vi "Lian_Conditional_Statistics.vi"() -> ()   [LabVIEW 2020]
uses:
  <vilib>/numeric/Random Number (Range) U64.vi
  <vilib>/numeric/sub_Random U32.vi
  <vilib>/Analysis/NI_AALBase.lvlib
panel:
  out "Final Array":u64[](array[numeric])
  out "Histogram":T1(graph)
  out "Mean":dbl
  out "Std Dev":dbl
  out "Final Array Size":i32
  out "Iteration Count":i32
  in  "Array Length":i32=100
  out "Final Array Size":i32
  out "Std Dev":dbl
  out "Mean":dbl
  out "FInal Array":dbl[](array[numeric])
  out "Histogram":T1(graph)
  in  "Array Length":i32=100
  in  "?":bool
  out "Iteration Count":i32
  out "Final Array Size":i32
  out "Iteration Count":i32
  out "Std Dev":dbl
  out "Mean":dbl
  out "FInal Array":dbl[](array[numeric])
  in  "?":bool
  out "Histogram":T1(graph)
  in  "Array Length":i32=100
  # "Conditional Statistics"
  # "Description: Filters data using logic and builds array"
  # "Conditional Statistics 3"
  # "Description:  Builds array with select data"
  # "Conditional Statistics 2"
  # "Description: Filters data using selector label and builds array"
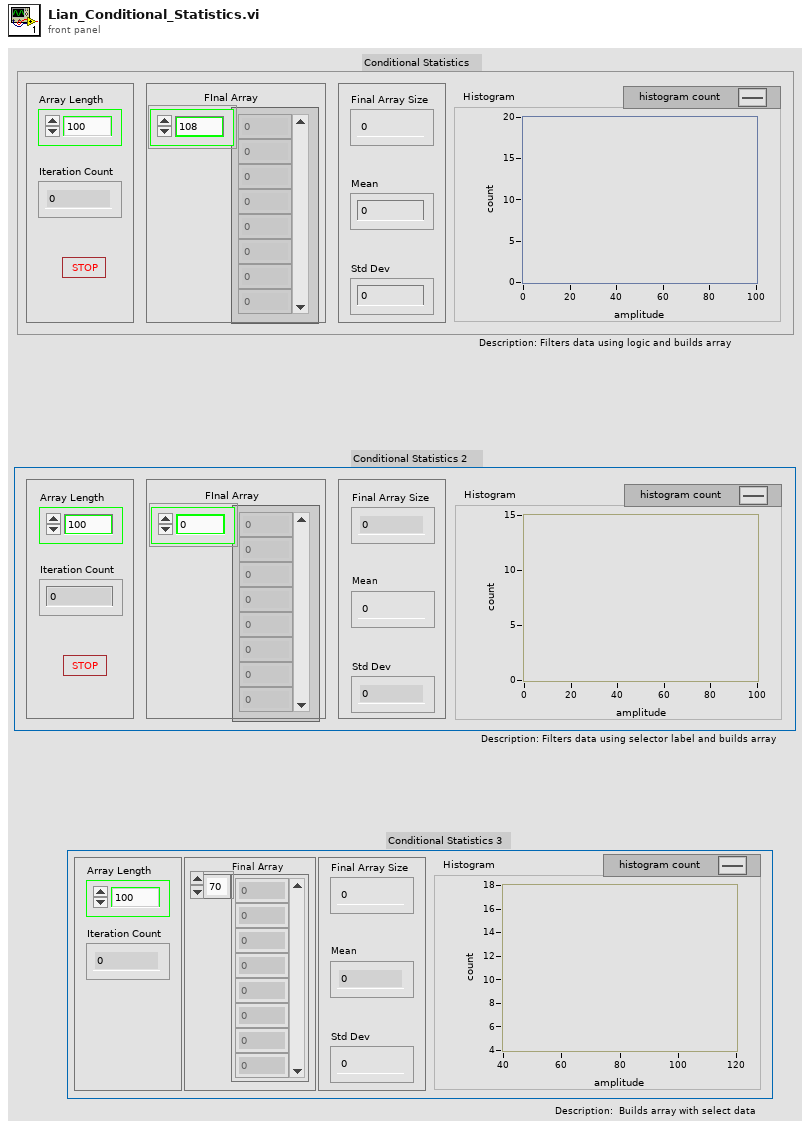
[diagram p1: front panel]
types:
  T1 = cluster{"X Values":dbl[], "Histogram: h(x)":i32[]}
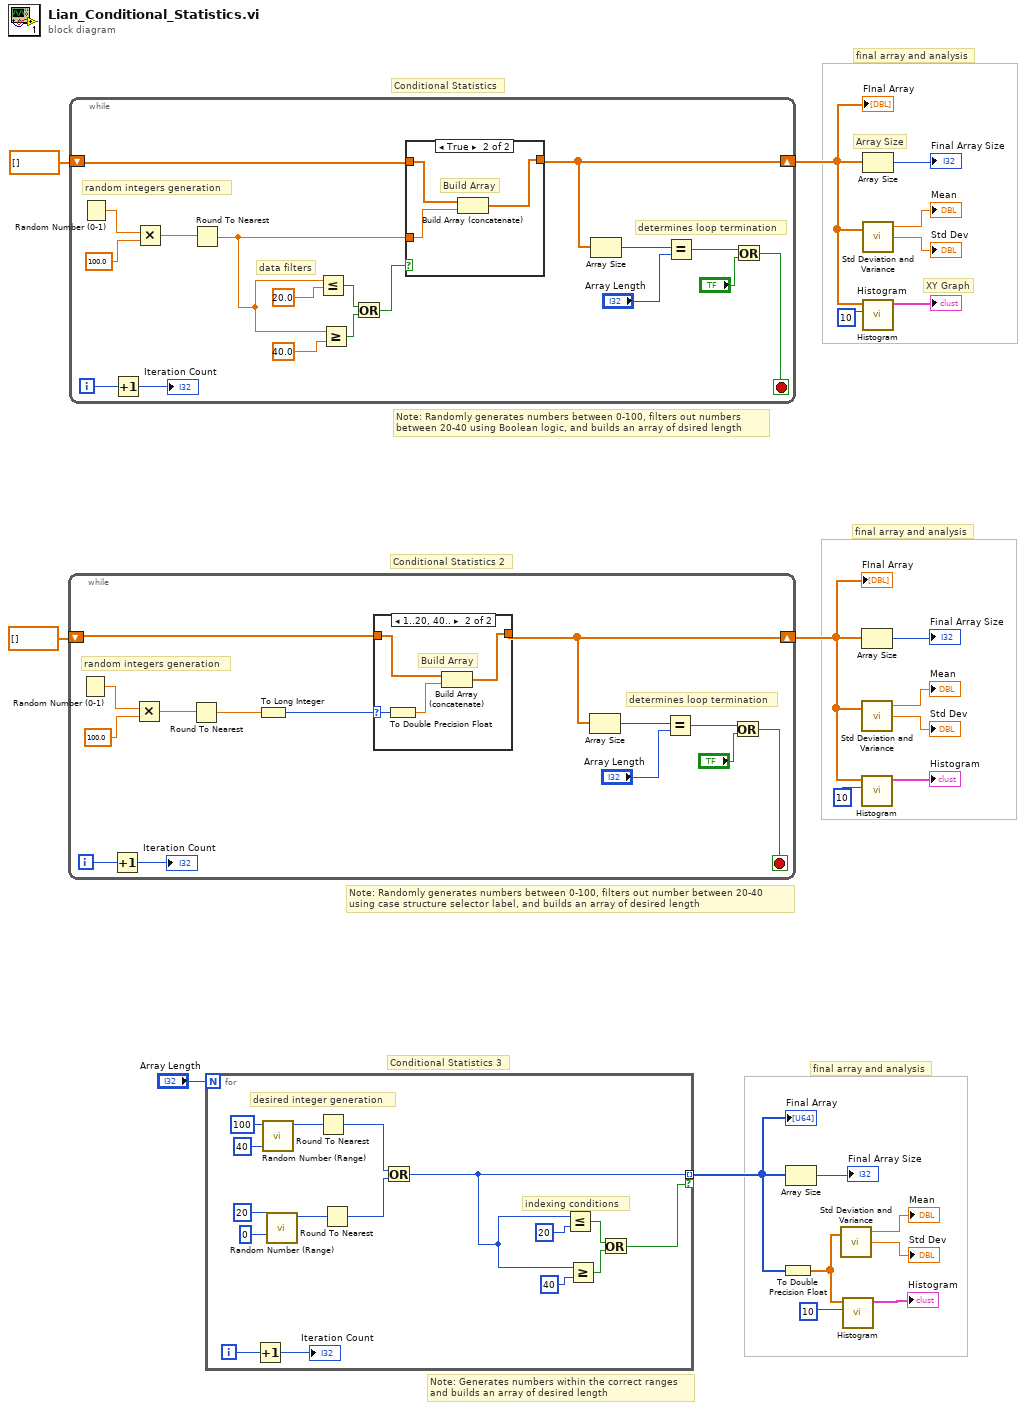
[diagram p0: block diagram]
diagram:
  # "Note: Generates numbers within the correct ranges\nand builds an array of desired length"
  # "Conditional Statistics 3"
  # "final array and analysis"
  # "Array Size"
  # "XY Graph"
  # "Note: Randomly generates numbers between 0-100, filters out number between 20-40 \nusing case structure selector label, and builds an array of desired length"
  # "Conditional Statistics 2"
  # "final array and analysis"
  # "Note: Randomly generates numbers between 0-100, filters out numbers \nbetween 20-40 using Boolean logic, and builds an array of dsired length"
  # "Conditional Statistics"
  # "final array and analysis"
  n1 = while {
    shift-right: [w28] -> w13
    shift-left: dbl[] [] -> [w29]
    i -> [w27]
    stop <- w33 stop-if-true
    # "determines loop termination"
    # "random integers generation"
    n2 = Random Number (0-1)() -> (number: 0 to 1=w36:dbl)
    n3 = Increment(x=w27) -> (x+1=→"Iteration Count":i32)
    n4 = Multiply(x=w36, y=100.0) -> (x*y=w34:dbl)
    n5 = Round To Nearest(number=w34) -> (nearest integer value=w24:dbl)
    n6 = To Long Integer(number=w24) -> (32bit integer=w23:i32)
    n7 = case shown="1..20, 40.." w23 {
      selector: w23 -> [_ w39]
      tunnel: w29 -> [w37 w41]
      tunnel: [w37 w40] -> w28
      frame 21..39, Default {
      }
      frame 1..20, 40.. {
        # "Build Array"
        n8 = To Double Precision Float(number=w39) -> (double precision float=w38:dbl)
        n9 = Build Array (concatenate)(w41, w38) -> (w40:dbl[])
      }
    }
    n10 = Array Size(array=w28) -> (size(s)=w32:i32)
    n11 = Equal?(x=w32, y="Array Length") -> (x = y?=w31:bool)
    n12 = Or(x=w31, y="?") -> (x .or. y?=w33:bool)
  }
  "FInal Array" <- w13
  n13 = while {
    shift-right: [w51] -> w20
    shift-left: dbl[] [] -> [w52]
    i -> [w44]
    stop <- w56 stop-if-true
    # "determines loop termination"
    # "random integers generation"
    # "data filters"
    n14 = Random Number (0-1)() -> (number: 0 to 1=w59:dbl)
    n15 = Increment(x=w44) -> (x+1=→"Iteration Count":i32)
    n16 = Multiply(x=w59, y=100.0) -> (x*y=w57:dbl)
    n17 = Round To Nearest(number=w57) -> (nearest integer value=w47:dbl)
    n18 = Less Or Equal?(x=w47, y=20.0) -> (x <= y?=w50:bool)
    n19 = Greater Or Equal?(x=w47, y=40.0) -> (x >= y?=w49:bool)
    n20 = Or(x=w50, y=w49) -> (x .or. y?=w48:bool)
    n21 = case shown="True" w48 {
      tunnel: w47 -> [_ w63]
      tunnel: w52 -> [w60 w62]
      tunnel: [w60 w61] -> w51
      frame False {
      }
      frame True {
        # "Build Array"
        n22 = Build Array (concatenate)(w62, w63) -> (w61:dbl[])
      }
    }
    n23 = Array Size(array=w51) -> (size(s)=w55:i32)
    n24 = Equal?(x=w55, y="Array Length") -> (x = y?=w54:bool)
    n25 = Or(x=w54, y="?") -> (x .or. y?=w56:bool)
  }
  "FInal Array" <- w20
  n26 = for {
    N: "Array Length" -> [_]
    tunnel: [w66] -> w2 mode=indexing if=w75
    i -> [w79]
    # "indexing conditions"
    # "desired integer generation"
    n27 = Increment(x=w79) -> (x+1=→"Iteration Count":i32)
    n28 = call-poly <vilib>:"Random Number (Range).vi"("lower bound (0)"=u64 40, "upper bound (100)"=u64 100) -> ("number"=w71:u64)  [unwired: 9 in]
    n29 = call-poly <vilib>:"Random Number (Range).vi"("lower bound (0)"=u64 0, "upper bound (100)"=u64 20) -> ("number"=w72:u64)  [unwired: 9 in]
    n30 = Round To Nearest(number=w71) -> (nearest integer value=w73:u64)
    n31 = Round To Nearest(number=w72) -> (nearest integer value=w74:u64)
    n32 = Or(x=w73, y=w74) -> (x .or. y?=w66:u64)
    n33 = Less Or Equal?(x=w66, y=u64 20 ("x")) -> (x <= y?=w77:bool)
    n34 = Greater Or Equal?(x=w66, y=u64 40 ("x")) -> (x >= y?=w76:bool)
    n35 = Or(x=w77, y=w76) -> (x .or. y?=w75:bool)
  }
  "Final Array" <- w2
  n36 = To Double Precision Float(number=w2) -> (double precision float=w1:dbl[])
  n37 = Array Size(array=w2) -> (size(s)=→"Final Array Size":i32)
  n38 = call <vilib>:"Std Deviation and Variance.vi"("X"=w1) -> ("mean"=→"Mean":dbl, "standard deviation"=→"Std Dev":dbl)  [unwired: 1 in, 1 out]
  n39 = call <vilib>:"Histogram.vi"("intervals"=10, "X"=w1) -> ("Histogram Graph"=→"Histogram":T1)  [unwired: 6 in, 3 out]
  n40 = Array Size(array=w13) -> (size(s)=→"Final Array Size":i32)
  n41 = call <vilib>:"Std Deviation and Variance.vi"("X"=w13) -> ("mean"=→"Mean":dbl, "standard deviation"=→"Std Dev":dbl)  [unwired: 1 in, 1 out]
  n42 = call <vilib>:"Histogram.vi"("intervals"=10, "X"=w13) -> ("Histogram Graph"=→"Histogram":T1)  [unwired: 6 in, 3 out]
  n43 = Array Size(array=w20) -> (size(s)=→"Final Array Size":i32)
  n44 = call <vilib>:"Std Deviation and Variance.vi"("X"=w20) -> ("mean"=→"Mean":dbl, "standard deviation"=→"Std Dev":dbl)  [unwired: 1 in, 1 out]
  n45 = call <vilib>:"Histogram.vi"("intervals"=10, "X"=w20) -> ("Histogram Graph"=→"Histogram":T1)  [unwired: 6 in, 3 out]
